vi "SetColorDigitalToDigitalCtrl.vi"(5 "text color":u32(colorbox)=16860, 7 "bg color":u32(colorbox)=16860, 10 "number":dbl, 11 "ref string":refnum<vi>) -> ()   [LabVIEW 2018, in "Library-Ctrl.lvlib"]
uses:
  Library-Ctrl.lvlib
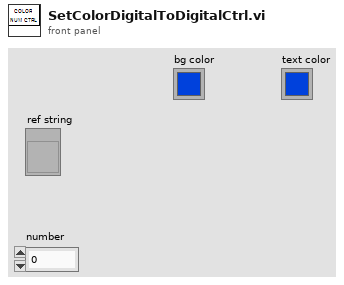
[diagram p1: front panel]
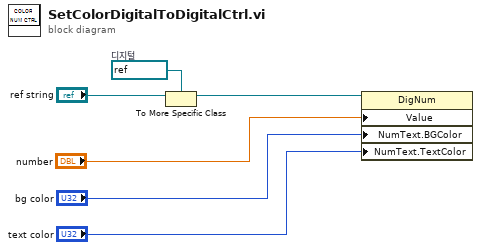
[diagram p0: block diagram]
diagram:
  w2 = refnum<vi> refnum  # 디지털
  n1 = To More Specific Class(target class=w2, reference="ref string") -> (specific class reference=w1:refnum<vi>)  [unwired: 1 in, 1 out]
  n2 = property class="DigNum"(reference=w1, "Value"="number", "NumText.BGColor"="bg color", "NumText.TextColor"="text color") -> ()  [unwired: 1 in, 2 out]
